vi "Read azVelocity.vi"(8 "error in (no error)":errorcluster, 11 "AzElTracking in":refnum<class "AzElTracking.lvclass">) -> (0 "error out":errorcluster, 2 "azVelocity":dbl[unit] min=-0.3490658503988659 max=0.3490658503988659, 3 "AzElTracking out":refnum<class "AzElTracking.lvclass">)   [LabVIEW 2022 SP3, in "TCSDataDefinitions.lvlib" / "TCSMountControlStatus.lvlib" / "AzElTracking.lvclass"]
uses:
  AzElTracking.lvclass
  AzElTracking.lvclass/AzElTracking.ctl
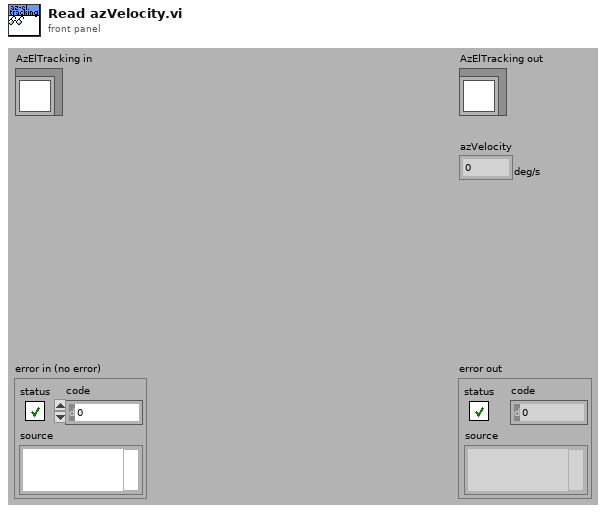
[diagram p1: front panel]
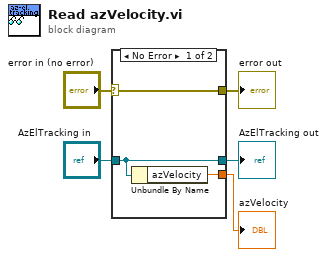
[diagram p0: block diagram]
diagram:
  n1 = case shown="No Error" "error in (no error)" {
    selector: "error in (no error)" -> [w8 w9]
    tunnel: [w8 w9] -> w4
    tunnel: [w7 w10] -> w2
    tunnel: "AzElTracking in" -> [w7 w10]
    tunnel: [w6 _] -> w1
    frame No Error {
      n2 = Unbundle By Name(w7) -> ("azVelocity"=w6:dbl[unit])
    }
    frame Error {
    }
  }
  "error out" <- w4
  "AzElTracking out" <- w2
  "azVelocity" <- w1
